vi "dfd_SCL_ARMANrmm_CU.vi"(8 "load":bool, 9 "global reset":bool, 11 "idx":u8) -> (3 "control signal":T1)   [LabVIEW 2017]
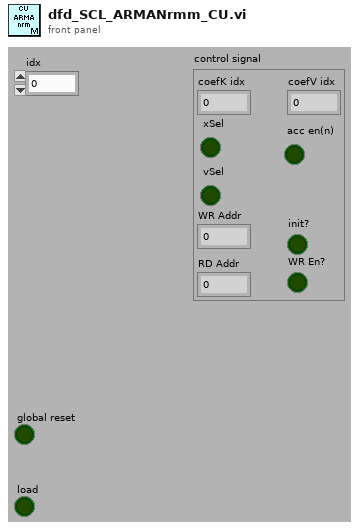
[diagram p1: front panel]
types:
  T1 = cluster{"coefK idx":u8, "coefV idx":u8, "xSel":bool, "vSel":bool, "acc en(n)":bool, "WR Addr":u16, "RD Addr":u16, "init?":bool, "WR En?":bool}
  T2 = cluster{"MEM RD Addr":u16, "MEM WR Addr":u16, "Ch cnt":u8, "first run?":bool}
  T3 = cluster{"coefK idx":u8, "coefV idx":u8, "xSel ctrl(n)":bool, "loop ctrl(n)":bool, "loop ctrl(n-1)":bool, "ySumSel ctrl(n)":bool, "ySumSel ctrl(n-1)":bool, "ySumSel ctrl(n-2)":bool, "ySumSel ctrl(n-3)":bool}
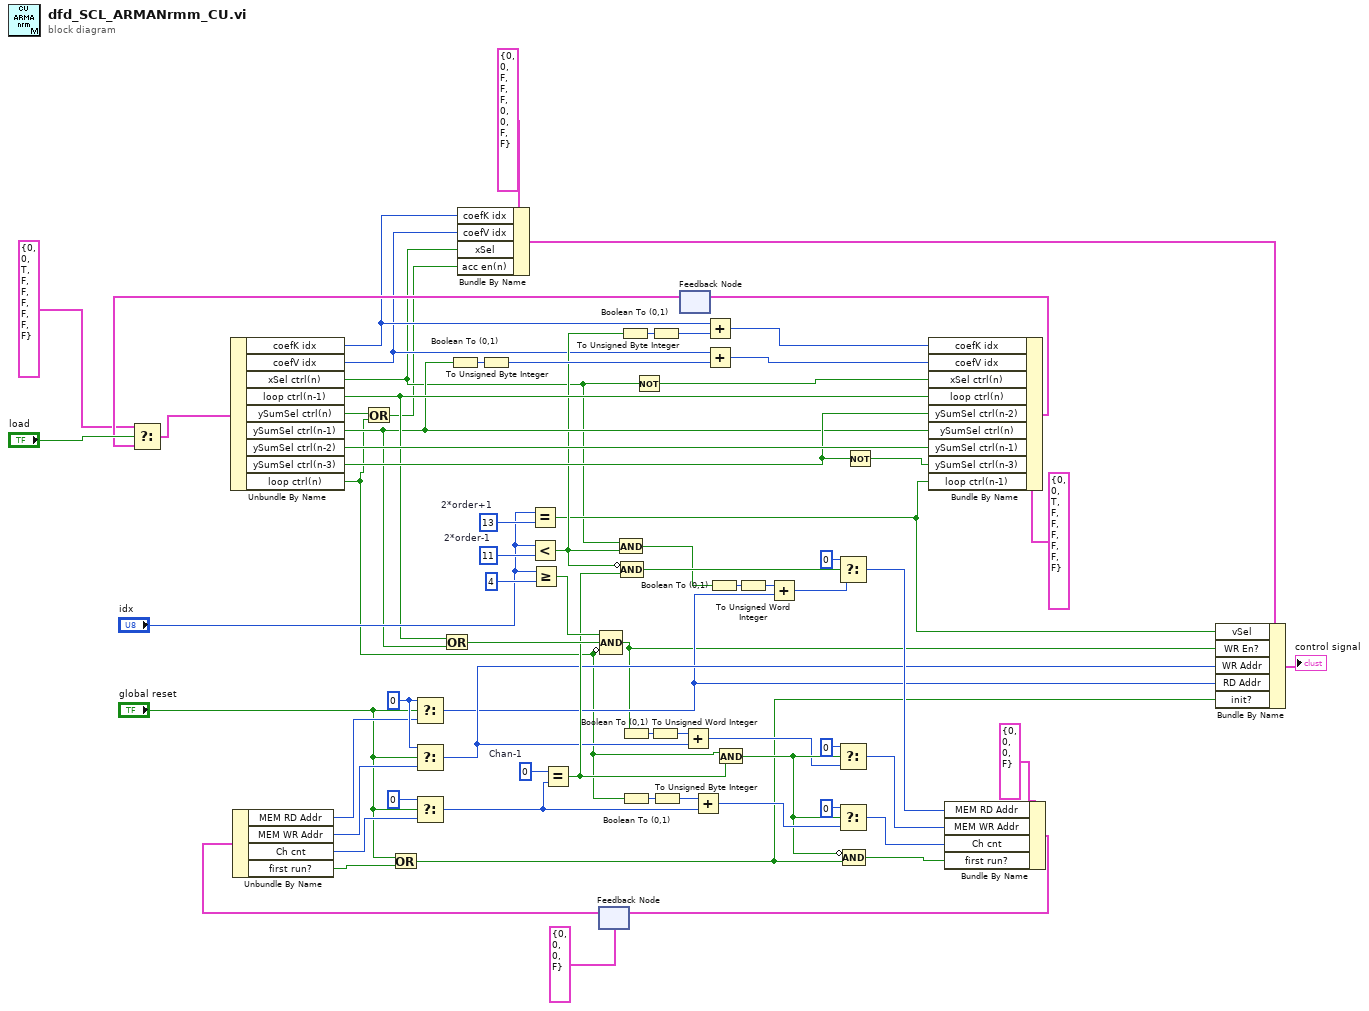
[diagram p0: block diagram]
diagram:
  w62 = u8 0  # Chan-1
  w70 = u16 0
  w71 = u8 11  # 2*order-1
  w72 = u8 13  # 2*order+1
  n1 = Equal?(x="idx", y=w72) -> (x = y?=w8:bool)
  n2 = Less?(x="idx", y=w71) -> (x < y?=w9:bool)
  n3 = Greater Or Equal?(x="idx", y=u8 4) -> (x >= y?=w50:bool)
  n4 = feedback #1(T2 {"MEM RD Addr"=0, "MEM WR Addr"=0, "Ch cnt"=0, "first run?"=FALSE} ("counter state in")) -> (w38:T2)
  n5 = Unbundle By Name(w38) -> ("MEM RD Addr"=w68:u16, "MEM WR Addr"=w67:u16, "Ch cnt"=w66:u8, "first run?"=w64:bool)
  n6 = Or(x="global reset", y=w64) -> (x .or. y?=w29:bool)
  n7 = Select(t=w70, s="global reset", f=w68) -> (s? t:f=w30:u16)
  n8 = Select(t=w70, s="global reset", f=w67) -> (s? t:f=w31:u16)
  n9 = Select(t=u8 0, s="global reset", f=w66) -> (s? t:f=w59:u8)
  n10 = Equal?(x=w62, y=w59) -> (x = y?=w46:bool)
  n11 = Boolean To (0,1)(Boolean=w9) -> (0, 1=w18:i16)
  n12 = Compound Arithmetic op=AND(invert w9, w46) -> (w45:bool)
  n13 = To Unsigned Byte Integer(number=w18) -> (unsigned 8bit integer=w17:u8)
  n14 = feedback #2() -> (w34:T3)  [unwired: 1 out]
  n15 = Select(t=T3 {"coefK idx"=0, "coefV idx"=0, "xSel ctrl(n)"=TRUE, "loop ctrl(n)"=FALSE, "loop ctrl(n-1)"=FALSE, "ySumSel ctrl(n)"=FALSE, "ySumSel ctrl(n-1)"=FALSE, "ySumSel ctrl(n-2)"=FALSE, "ySumSel ctrl(n-3)"=FALSE} ("control state out"), s="load", f=w34) -> (s? t:f=w12:T3)
  n16 = Unbundle By Name(w12) -> ("coefK idx"=w6:u8, "coefV idx"=w5:u8, "xSel ctrl(n)"=w4:bool, "loop ctrl(n-1)"=w11:bool, "ySumSel ctrl(n)"=w3:bool, "ySumSel ctrl(n-1)"=w10:bool, "ySumSel ctrl(n-2)"=w23:bool, "ySumSel ctrl(n-3)"=w22:bool, "loop ctrl(n)"=w1:bool)
  n17 = Or(x=w3, y=w1) -> (x .or. y?=w2:bool)
  n18 = Or(x=w11, y=w10) -> (x .or. y?=w51:bool)
  n19 = Boolean To (0,1)(Boolean=w10) -> (0, 1=w21:i16)
  n20 = Bundle By Name(cluster=T1 {"coefK idx"=0, "coefV idx"=0, "xSel"=FALSE, "vSel"=FALSE, "acc en(n)"=FALSE, "WR Addr"=0, "RD Addr"=0, "init?"=FALSE, "WR En?"=FALSE} ("control signal"), "coefK idx"=w6, "coefV idx"=w5, "xSel"=w4, "acc en(n)"=w2) -> (w26:T1)
  n21 = To Unsigned Byte Integer(number=w21) -> (unsigned 8bit integer=w20:u8)
  n22 = Compound Arithmetic op=AND(w50, w51, invert w1) -> (w28:bool)
  n23 = And(x=w4, y=w9) -> (x .and. y?=w39:bool)
  n24 = Boolean To (0,1)(Boolean=w28) -> (0, 1=w48:i16)
  n25 = Boolean To (0,1)(Boolean=w1) -> (0, 1=w61:i16)
  n26 = Not(x=w4) -> (.not. x?=w15:bool)
  n27 = To Unsigned Word Integer(number=w48) -> (unsigned 16bit integer=w49:u16)
  n28 = To Unsigned Byte Integer(number=w61) -> (unsigned 8bit integer=w60:u8)
  n29 = Add(x=w49, y=w31) -> (x+y=w47:u16)
  n30 = Add(x=w60, y=w59) -> (x+y=w57:u8)
  n31 = Add(x=w6, y=w17) -> (x+y=w16:u8)
  n32 = Add(x=w5, y=w20) -> (x+y=w19:u8)
  n33 = Boolean To (0,1)(Boolean=w39) -> (0, 1=w41:i16)
  n34 = And(x=w1, y=w46) -> (x .and. y?=w54:bool)
  n35 = To Unsigned Word Integer(number=w41) -> (unsigned 16bit integer=w40:u16)
  n36 = Add(x=w40, y=w30) -> (x+y=w43:u16)
  n37 = Select(t=u16 0, s=w45, f=w43) -> (s? t:f=w42:u16)
  n38 = Select(t=u16 0, s=w54, f=w47) -> (s? t:f=w53:u16)
  n39 = Select(t=u8 0, s=w54, f=w57) -> (s? t:f=w56:u8)
  n40 = Compound Arithmetic op=AND(invert w54, w29) -> (w63:bool)
  n41 = Not(x=w22) -> (.not. x?=w24:bool)
  n42 = Bundle By Name(cluster=T3 {"coefK idx"=0, "coefV idx"=0, "xSel ctrl(n)"=TRUE, "loop ctrl(n)"=FALSE, "loop ctrl(n-1)"=FALSE, "ySumSel ctrl(n)"=FALSE, "ySumSel ctrl(n-1)"=FALSE, "ySumSel ctrl(n-2)"=FALSE, "ySumSel ctrl(n-3)"=FALSE} ("control state out"), "coefK idx"=w16, "coefV idx"=w19, "xSel ctrl(n)"=w15, "loop ctrl(n)"=w11, "ySumSel ctrl(n-2)"=w22, "ySumSel ctrl(n)"=w10, "ySumSel ctrl(n-1)"=w23, "ySumSel ctrl(n-3)"=w24, "loop ctrl(n-1)"=w8) -> (w14:T3)
  n43 = feedback-in #2(w14) -> ()
  n44 = Bundle By Name(cluster=T2 {"MEM RD Addr"=0, "MEM WR Addr"=0, "Ch cnt"=0, "first run?"=FALSE} ("counter state in"), "MEM RD Addr"=w42, "MEM WR Addr"=w53, "Ch cnt"=w56, "first run?"=w63) -> (w36:T2)
  n45 = feedback-in #1(w36) -> ()
  n46 = Bundle By Name(cluster=w26, "vSel"=w8, "WR En?"=w28, "WR Addr"=w31, "RD Addr"=w30, "init?"=w29) -> (→"control signal":T1)
